vi "Measurement UI.vi"() -> ()   [LabVIEW 2021, in "Crosstalk_Audio DAC_UI.lvlib"]
uses:
  Crosstalk_Audio DAC_UI.lvlib
  shared/audio popup ui/Audio Popup UI.lvlib
  Crosstalk_Audio DAC.lvlib
panel:
  out "Time domain graph":waveform(dbl)[](graph)
  out "Frequency domain graph":cluster{"f0":dbl, "df":dbl, dbl[]}[](graph)
  out "Table results":string[][](table)
  in  "settings tab":T1(tab)
  in  "Interferrer channel":u32 caption="INTERFERRER CHANNEL"
  in  "Interferrer channel resource":string caption="INTERFERRER CHANNEL RESOURCE"
  in  "Min settling time (s)":dbl=0.1 caption="MINIMUM SETTLING TIME" format="%#_6ps"
  in  "Min settling cycles":u32 caption="MINIMUM SETTLING CYCLES"
  in  "Min measurement time (s)":dbl=0.1 caption="MINIMUM MEASUREMENT TIME" format="%#_6ps"
  in  "Min measurement cycles":u32 caption="MINIMUM MEASUREMENT CYCLES"
  in  "Sample rate (Hz)":dbl=51200.0 caption="SAMPLE RATE" format="%#_6pHz"
  in  "Victim channel resource":string caption="VICTIM CHANNEL RESOURCE"
  in  "Output range (Vpk-pk)":dbl=15.0 caption="OUTPUT RANGE" format="%.3p Vpk-pk"
  in  "Output level units":string(combo)="dBFS" caption="SNR"
  in  "Output level":dbl=-1.0 caption="OUTPUT LEVEL" format="%#_6p"
  in  "Frequency (Hz)":dbl=1000.0 caption="FREQUENCY" format="%#_6pHz"
  in  "Master clock channel":string caption="MASTER CLOCK CHANNEL"
  in  "Digital audio channel":string caption="DIGITAL AUDIO CHANNEL"
  out "digital serial file name":string
  in  "configure digital serial":bool
  in  "Band stop (Hz)":dbl=20000.0 caption="BAND STOP" format="%#_6pHz"
  in  "Band start (Hz)":dbl=20.0 caption="BAND START" format="%#_6pHz"
  in  "Weighting filter":string(combo)="A-weighting" caption="WEIGHTING FILTER"
  in  "Lowpass filter":string(combo)="No filter" caption="LOWPASS FILTER"
  in  "Highpass filter":string(combo)="DC" caption="HIGHPASS FILTER"
  out "Crosstalk":dbl[](array[numeric]) format="%_6g"
  out "Frequency":dbl[](array[numeric]) format="%_6g"
  out "df":dbl format="%_6g"
  out "f0":dbl format="%_6g"
  out "dt":dbl format="%_6g"
  out "Frequency domain":dbl[](array[numeric]) format="%_6g"
  out "Time domain":dbl[](array[numeric]) format="%_6g"
  out "Channel names":string[](array[string])
  in  "Protocol file":string
  # "Protocol settings"
  # "Generation settings"
  # "Acquisition settings"
  # "Filters"
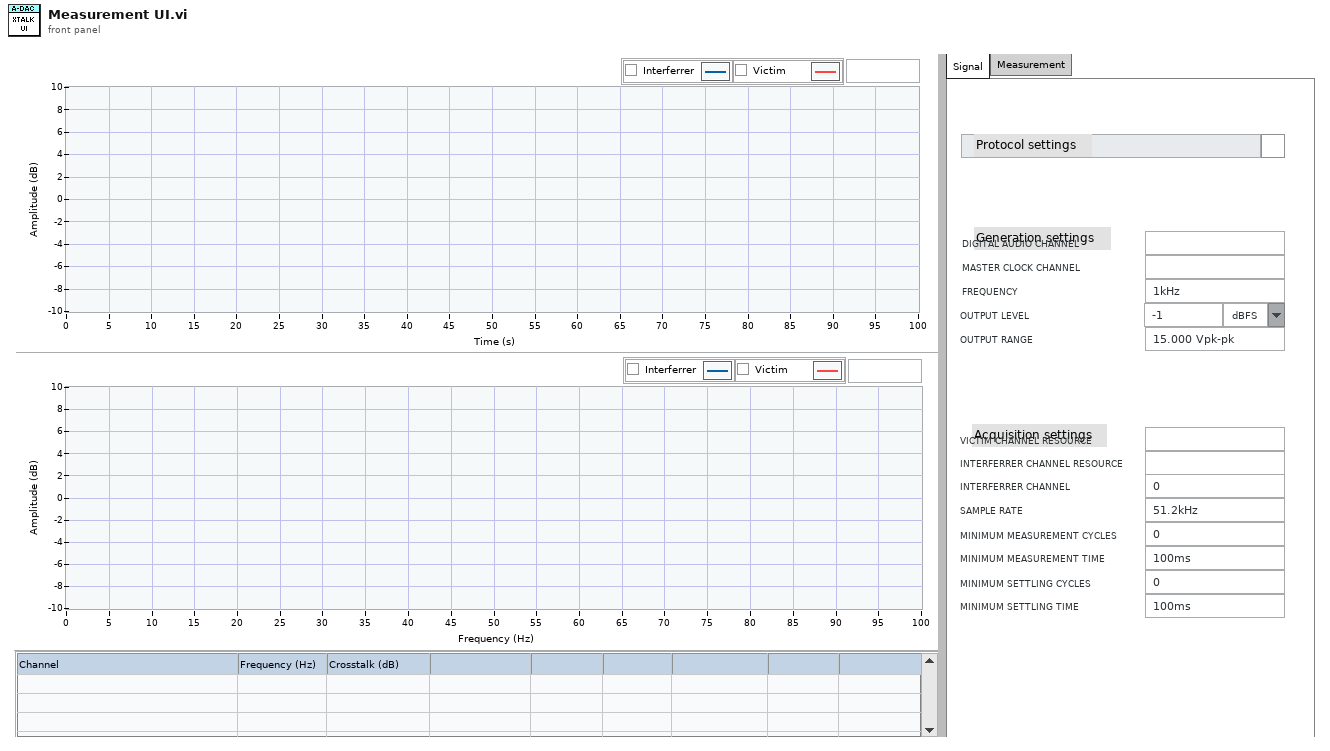
[diagram p1: front panel]
types:
  T1 = enum32{"Signal", "Measurement", "HiddenControls"}
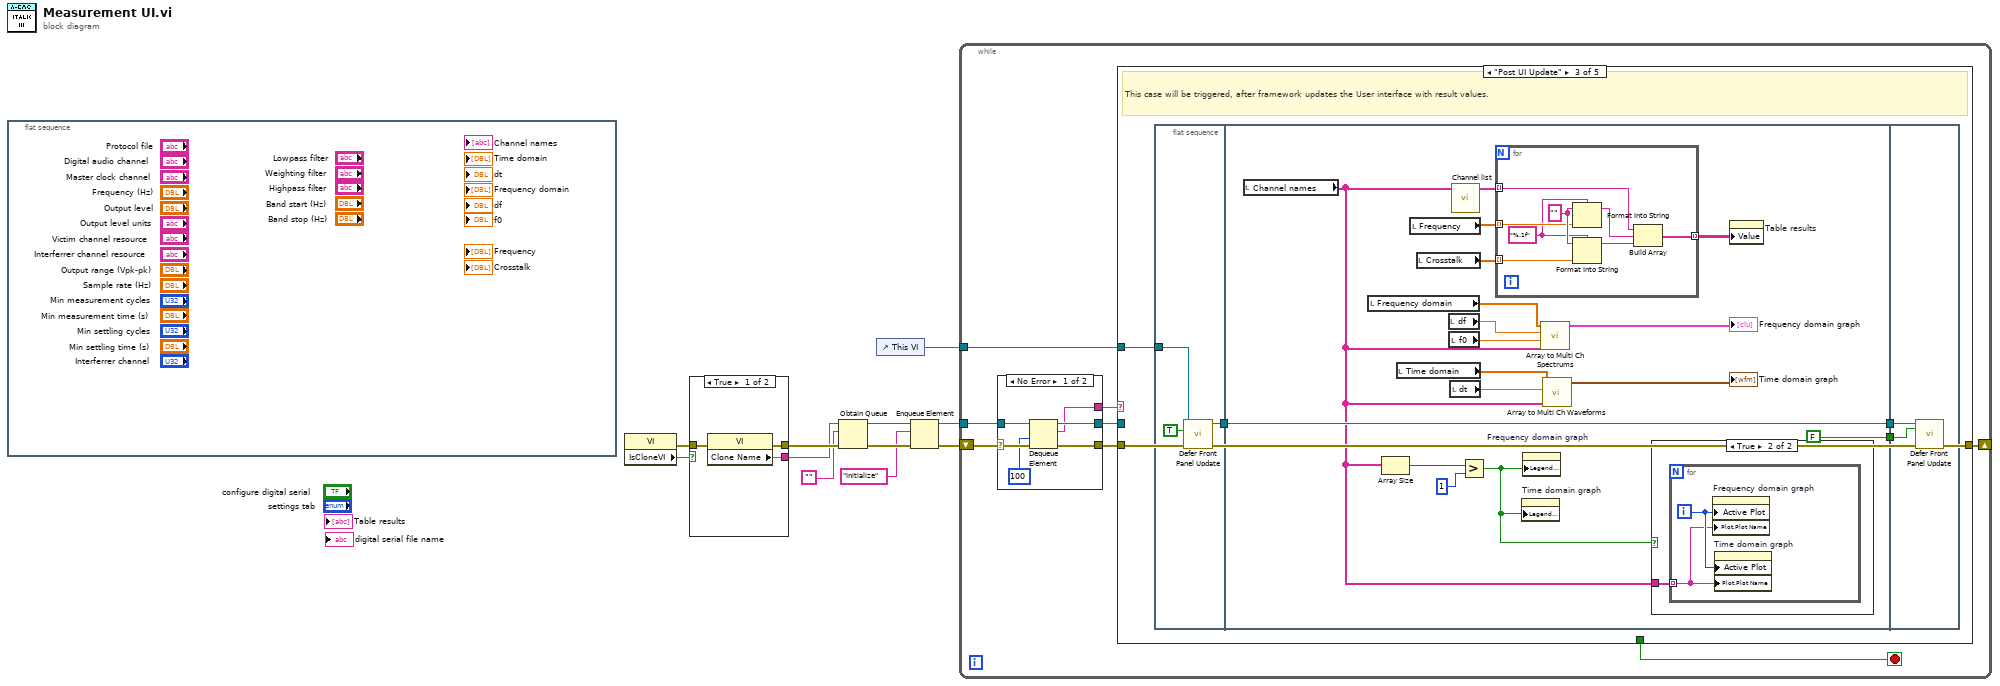
[diagram p0: block diagram]
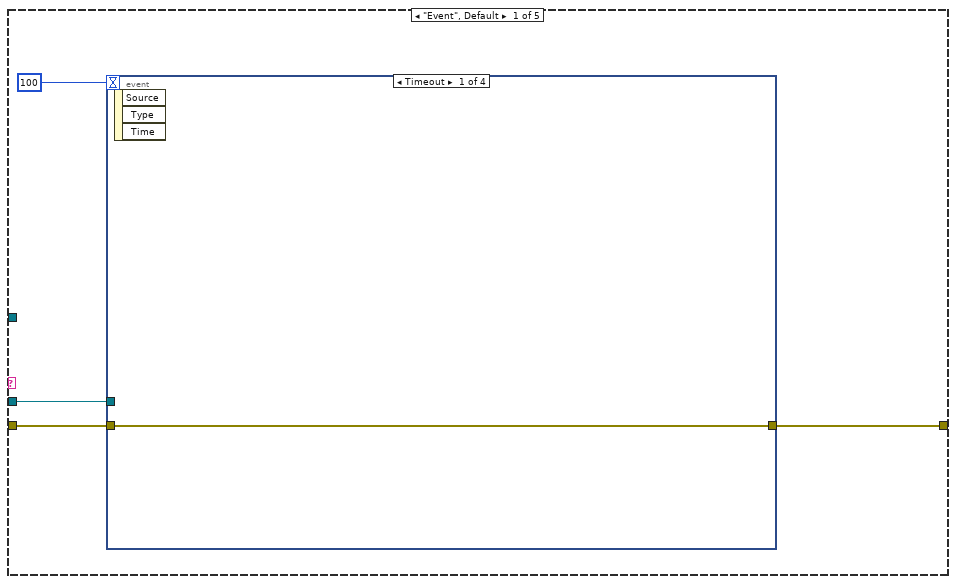
[diagram p2: hidden frame]
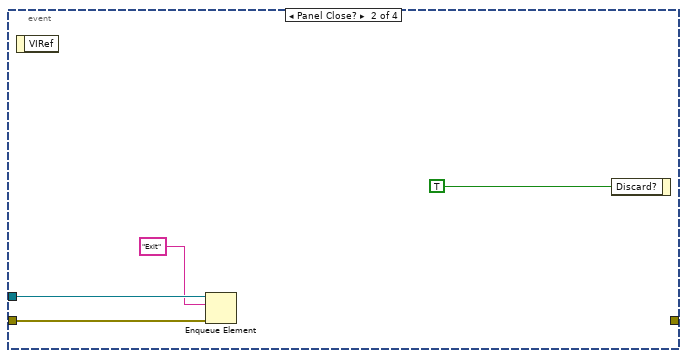
[diagram p3: hidden frame]
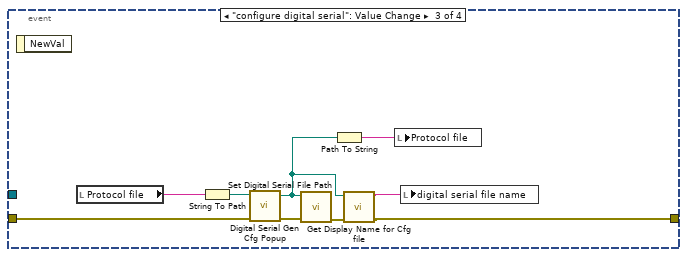
[diagram p4: hidden frame]
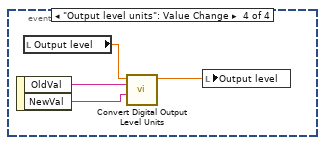
[diagram p5: hidden frame]
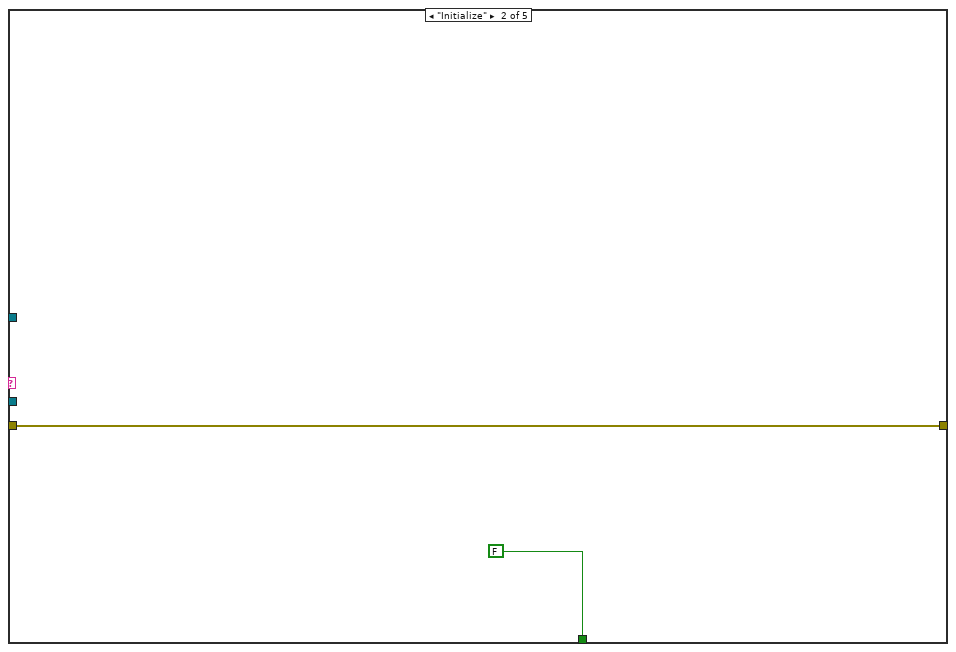
[diagram p6: hidden frame]
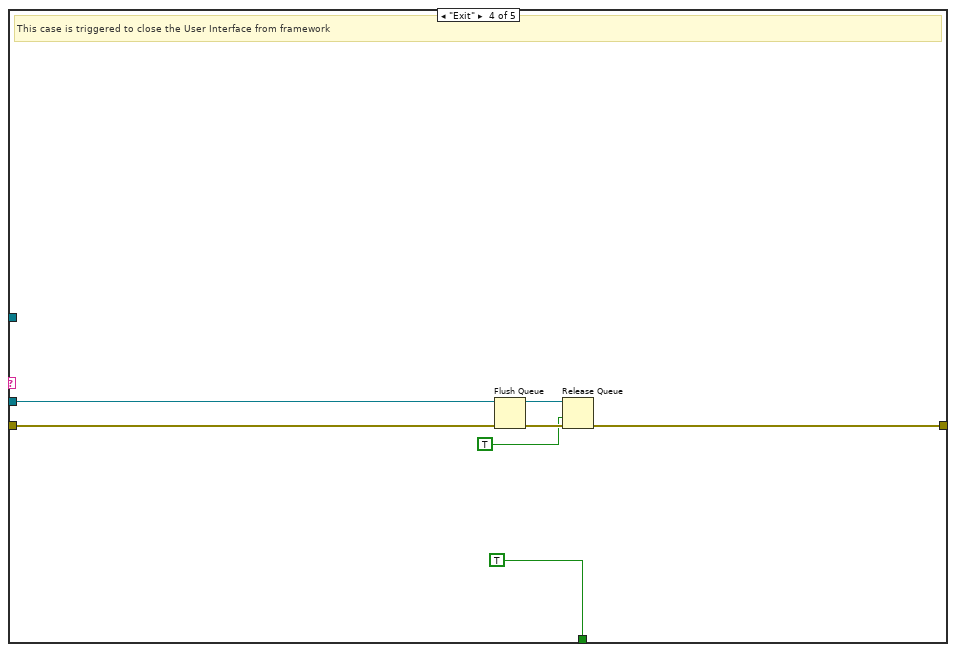
[diagram p8: hidden frame]
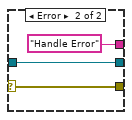
[diagram p10: hidden frame]
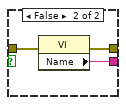
[diagram p11: hidden frame]
diagram:
  n1 = flat-sequence {
    frame #0 {
    }
  }
  n2 = property class="VI"() -> (error out=w2:errorcluster, "IsCloneVI"=w3:bool)  [unwired: 2 in, 1 out]
  n3 = case shown="True" w3 {
    tunnel: [w14 w17] -> w11
    tunnel: [w13 w16] -> w10
    tunnel: w2 -> [w12 w15]
    frame True {
      n4 = property class="VI"(error in=w12) -> (error out=w14:errorcluster, "Clone Name"=w13:string)  [unwired: 1 in, 1 out]
    }
    frame False {
      n5 = property class="VI"(error in=w15) -> (error out=w17:errorcluster, "Name"=w16:string)  [unwired: 1 in, 1 out]
    }
  }
  n6 = Obtain Queue(name (unnamed)=w10, element data type="", error in (no error)=w11) -> (queue out=w7:refnum<queue>, error out=w9:errorcluster)  [unwired: 2 in, 1 out]
  n7 = control-ref of="This VI"() -> (w1:refnum<vi>)
  n8 = Enqueue Element(queue=w7, element="Initialize", error in (no error)=w9) -> (queue out=w6:refnum<queue>, error out=w8:errorcluster)  [unwired: 1 in, 1 out]
  n9 = while {
    shift-right: [w20] -> _
    shift-left: w8 -> [w25]
    tunnel: w6 -> [w23]
    tunnel: w1 -> [w18]
    stop <- w19 stop-if-true
    n10 = case shown="No Error" w25 {
      selector: w25 -> [w101 w104]
      tunnel: [w100 w104] -> w24
      tunnel: w23 -> [w99 w103]
      tunnel: [w98 w103] -> w22
      tunnel: [w97 "Handle Error"] -> w21
      frame No Error {
        n11 = Dequeue Element(queue=w99, timeout in ms (-1)=100, error in (no error)=w101) -> (queue out=w98:refnum<queue>, element=w97:string, error out=w100:errorcluster)  [unwired: 1 out]
      }
      frame Error {
      }
    }
    n12 = case shown="\"Post UI Update\"" w21 {
      tunnel: w24 -> [w28 w49 w54 w94 w95]
      tunnel: w22 -> [w26 _ _ w92 _]
      tunnel: [w29 w49 w54 w89 w95] -> w20
      tunnel: [_ FALSE _ TRUE _] -> w19
      tunnel: w18 -> [_ _ w53 _ _]
      frame "Event", Default {
        n13 = event shown="[0] Timeout" {
          selector: _ -> [_ _ _ _]
          dyn-events: _ -> [_ _ _ _]
          timeout: 100 -> [_ _ _ _]
          tunnel: [w30 _ w35 _] -> w29
          tunnel: w28 -> [w30 w33 w40 _]
          tunnel: w26 -> [_ w32 _ _]
          event Timeout {
            n14 = event-data() -> ()  [unwired: 1 in, 3 out]
          }
          event Panel Close? {
            n15 = event-data() -> ()  [unwired: 1 in, 1 out]
            n16 = Enqueue Element(queue=w32, element="Exit", error in (no error)=w33) -> ()  [unwired: 1 in, 3 out]
            n17 = event-data("Discard?"=TRUE) -> ()  [unwired: 1 in, 1 out]
          }
          event "configure digital serial": Value Change {
            n18 = event-data() -> ()  [unwired: 1 in, 1 out]
            n19 = local read "Protocol file"() -> (w43:string)
            n20 = String To Path(string=w43) -> (path=w41:path)
            n21 = call "Digital Serial Gen Cfg Popup.vi"("error in (no error)"=w40, "config file in"=w41) -> ("error out"=w39:errorcluster, "config file out"=w37:path)  [unwired: 7 in, 1 out]
            n22 = call "Set Digital Serial File Path.vi"("error in (no error)"=w39, "digital serial file"=w37) -> ("error out"=w38:errorcluster)  [unwired: 9 in]
            n23 = Path To String(path=w37) -> (string=w42:string)
            n24 = call "Get Display Name for Cfg file.vi"("error in (no error)"=w38, "file path"=w37) -> ("error out"=w35:errorcluster, "display string"=w36:string)  [unwired: 8 in]
            n25 = local write "Protocol file"(w42) -> ()
            n26 = local write "digital serial file name"(w36) -> ()
          }
          event "Output level units": Value Change {
            n27 = event-data() -> ("OldVal"=w47:string, "NewVal"=w46:string)  [unwired: 1 in]
            n28 = local read "Output level"() -> (w45:dbl)
            n29 = call "Convert Digital Output Level Units.vi"("New output level units"=w46, "Previous output level units"=w47, "Previous output level"=w45) -> ("New output level"=w44:dbl)  [unwired: 8 in]
            n30 = local write "Output level"(w44) -> ()
          }
        }
      }
      frame "Initialize" {
      }
      frame "Post UI Update" {
        # "This case will be triggered, after framework updates the User interface with result values."
        n31 = flat-sequence {
          tunnel: w53 -> [w57]
          tunnel: [w55] -> w51
          tunnel: [w65] -> w52
          tunnel: w51 -> [w65]
          tunnel: [FALSE] -> w50
          tunnel: w52 -> [w87]
          tunnel: w50 -> [w86]
          frame #0 {
            n32 = call "Defer Front Panel Update.vi"("Defer Panel Updates"=TRUE, "VI in"=w57) -> ("VI out"=w55:refnum<vi>)  [unwired: 8 in, 1 out]
          }
          frame #1 {
            n33 = local read "Channel names"() -> (w58:string[])
            n34 = local read "Frequency domain"() -> (w74:dbl[])
            n35 = Array Size(array=w58) -> (size(s)=w61:i32)
            n36 = local read "Time domain"() -> (w71:dbl[])
            n37 = local read "Frequency"() -> (w67:dbl[])
            n38 = local read "Crosstalk"() -> (w66:dbl[])
            n39 = local read "df"() -> (w73:dbl)
            n40 = local read "f0"() -> (w72:dbl)
            n41 = local read "dt"() -> (w70:dbl)
            n42 = call "Channel list.vi"("Channel list"=w58) -> ("channel names"=w62:string[])  [unwired: 10 in]
            n43 = Greater?(x=w61, y=1) -> (0:w59:bool)
            n44 = for {
              tunnel: w67 -> [w84] mode=indexing
              tunnel: w66 -> [w83] mode=indexing
              tunnel: [w80] -> w63 mode=indexing
              tunnel: w62 -> [w79] mode=indexing
              w78 = "%.1f" ("format string")
              w85 = ""
              n45 = Format Into String(format string=w78, initial string=w85, w84) -> (resulting string=w82:string)  [unwired: 1 in, 1 out]
              n46 = Format Into String(format string=w78, initial string=w85, w83) -> (resulting string=w81:string)  [unwired: 1 in, 1 out]
              n47 = Build Array(w79, w82, w81) -> (w80:string[])
            }
            n48 = property on="Time domain graph" class="WFGraph (strict)"("Legend Visible"=w59) -> ()  [unwired: 2 in, 2 out]
            n49 = property on="Frequency domain graph" class="WFGraph (strict)"("Legend Visible"=w59) -> ()  [unwired: 2 in, 2 out]
            n50 = call "Array to Multi Ch Spectrums.vi"("channel names"=w58, "f0"=w72, "df"=w73, "array"=w74) -> ("spectra"=→"Frequency domain graph":cluster{"x0":dbl, "dx":dbl, "magnitude":dbl[]}[])  [unwired: 7 in]
            n51 = call "Array to Multi Ch Waveforms.vi"("channel names"=w58, "dt"=w70, "array"=w71) -> ("waveforms"=→"Time domain graph":waveform(dbl)[])  [unwired: 8 in]
            n52 = case shown="True" w59 {
              tunnel: w58 -> [_ w75]
              frame False {
              }
              frame True {
                n53 = for {
                  tunnel: w75 -> [w76] mode=indexing
                  i -> [w77]
                  n54 = property on="Frequency domain graph" class="WFGraph (strict)"("Active Plot"=w77, "Plot.Plot Name"=w76) -> ()  [unwired: 2 in, 2 out]
                  n55 = property on="Time domain graph" class="WFGraph (strict)"("Active Plot"=w77, "Plot.Plot Name"=w76) -> ()  [unwired: 2 in, 2 out]
                }
              }
            }
            n56 = property on="Table results" class="Tbl (strict)"("Value"=w63) -> ()  [unwired: 2 in, 2 out]
          }
          frame #2 {
            n57 = call "Defer Front Panel Update.vi"("Defer Panel Updates"=w86, "VI in"=w87) -> ()  [unwired: 8 in, 2 out]
          }
        }
      }
      frame "Exit" {
        # "This case is triggered to close the User Interface from framework"
        n58 = Flush Queue(queue=w92, error in (no error)=w94) -> (queue out=w91:refnum<queue>, error out=w90:errorcluster)  [unwired: 1 out]
        n59 = Release Queue(queue=w91, force destroy? (F)=TRUE, error in (no error)=w90) -> (error out=w89:errorcluster)  [unwired: 2 out]
      }
      frame "Handle Error" {
      }
    }
  }
